vi "AIs-Freq_CA.vi"(5 "下限值":dbl=1.7 format="%#_13g", 6 "Slot":T1, 7 "上限值":dbl=3.0 format="%#_13g", 8 "error in":errorcluster, 9 "循环次数":i32=10, 10 "Mode":string, 11 "CHs":string[](array[string])) -> (0 "error out":errorcluster, 1 "幅值":dbl caption="检测到的幅值" format="%.2p", 2 "RMS value":dbl caption="均方根值" format="%0.2p", 3 "波形图":waveform(dbl)[](graph), 4 "Strout":string)   [LabVIEW 2013]
uses:
  SystemCode/SysControl/Slot.ctl
  <vilib>/Analysis/3filter.llb/Filter Passband Type.ctl
  <vilib>/DAQmx/read.llb/DAQmx Read (Analog 1D Wfm NChan NSamp).vi
  SourceCode/GlobalValue.vi
  <vilib>/DAQmx/create/channels.llb/DAQmx Create Channel (AI-Voltage-Basic).vi
  <vilib>/DAQmx/configure/timing.llb/DAQmx Timing (Sample Clock).vi
  <vilib>/Analysis/3filter.llb/Butterworth Filter (DBL).vi
  <vilib>/measure/matone.llb/Extract Single Tone Information 1 Chan.vi
  <vilib>/measure/matone.llb/SINAD Analyzer 1 Chan.vi
  <vilib>/measure/madcrms.llb/Basic Averaged DC-RMS for 1 Chan.vi
  <vilib>/DAQmx/miscellaneous.llb/DAQmx Fill In Error Info.vi
  <vilib>/measure/NI_MAPro.lvlib
  <vilib>/Analysis/NI_AALBase.lvlib
panel:
  out "THD Plus Noise":dbl caption="总谐波失真叠加噪声" format="%.2p"
  out "SINAD (dB)":dbl format="%.2p"
  # "ASelfTest"
  # "Audio"
  # "Audio"
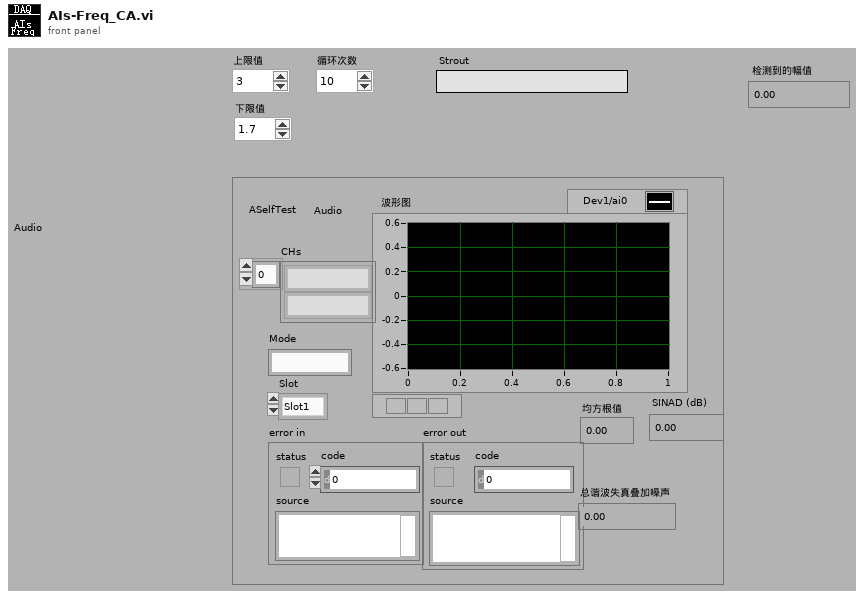
[diagram p1: front panel]
types:
  T1 = typedef "Slot.ctl" = enum16{"Slot1", "Slot2", "Slot3", "Slot4"}
  T2 = typedef "NI_AALBase.lvlib/Filter Passband Type.ctl" = enum32{"Lowpass", "Highpass", "Bandpass", "Bandstop"}
  T3 = typedef "DAQConfig.ctl" = cluster{"DIO":string[][], "AO":string[][], "AI":string[][]}
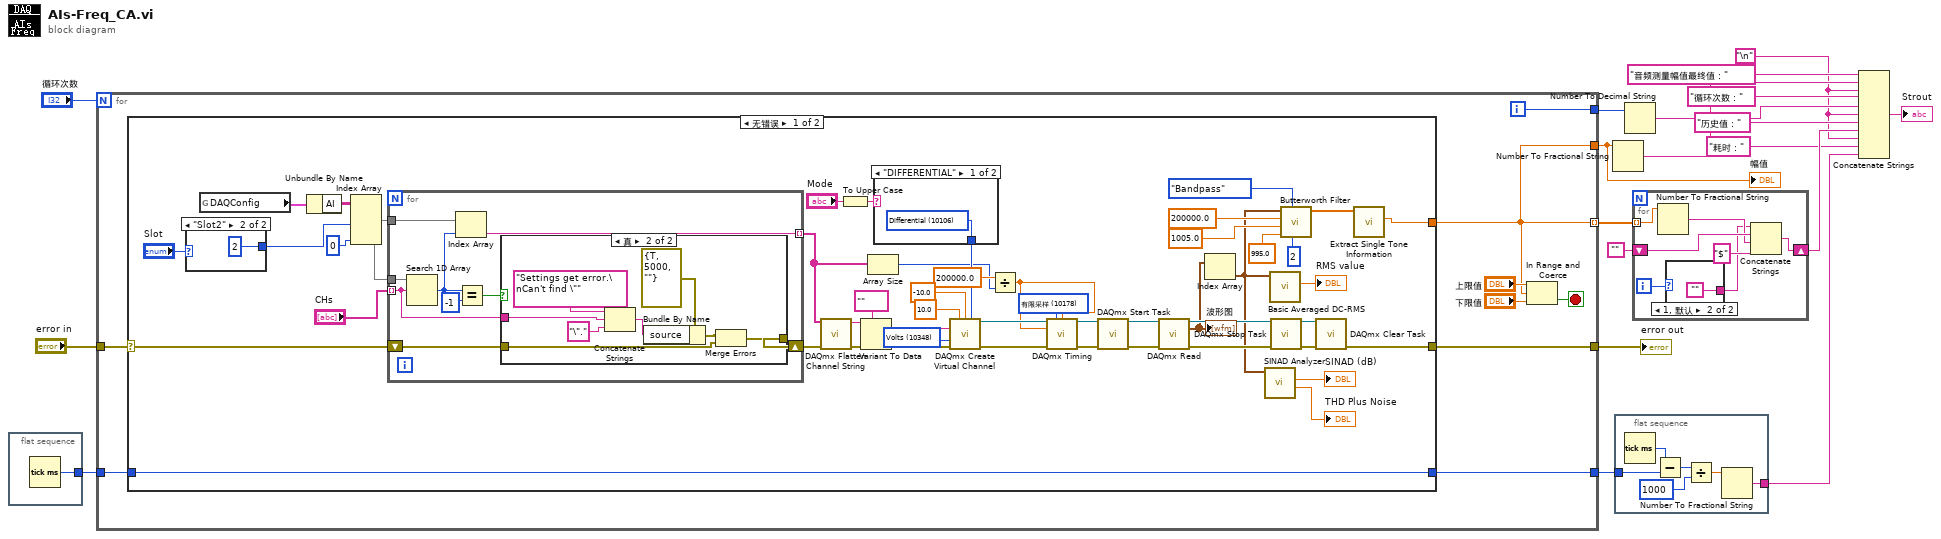
[diagram p0: block diagram]
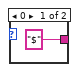
[diagram p2: hidden frame]
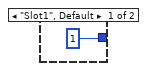
[diagram p3: hidden frame]
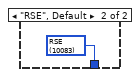
[diagram p5: hidden frame]
diagram:
  w5 = "\n"
  n1 = flat-sequence {
    tunnel: [w20] -> w18
    frame #0 {
      n2 = Tick Count (ms)() -> (millisecond timer value=w20:u32)
    }
  }
  n3 = for {
    N: "循环次数" -> [_]
    tunnel: [w22] -> w9 mode=indexing
    tunnel: w18 -> [w29]
    tunnel: [w28] -> w17
    tunnel: [w24] -> w16
    tunnel: "error in" -> [w23]
    tunnel: [w22] -> w1
    tunnel: [w21] -> w11
    i -> [w21]
    stop <- w27 stop-if-true
    n4 = case shown="无错误" w23 {
      selector: w23 -> [w63 w103]
      tunnel: [w79 w103] -> w24
      tunnel: [w38 _] -> w22
      tunnel: w29 -> [w37 w102]
      tunnel: [w37 w102] -> w28
      frame No Error {
        w59 = 10178 items=["有限采样"=10178, "连续采样"=10123, "硬件定时单点"=12522] ("sample mode")
        w74 = 10348 items=["Volts"=10348, "From Custom Scale"=10065] ("units")
        n5 = case shown="\"Slot2\"" "Slot" {
          tunnel: [1 ("索引 (行)") 2 ("索引 (行)")] -> w45
          frame "Slot1", Default {
          }
          frame "Slot2" {
          }
        }
        n6 = global read "GlobalValue.vi" "DAQConfig"() -> (w43:T3)
        n7 = Unbundle By Name(w43) -> ("AI"=w70:string[][])
        n8 = Index Array(array=w70, index (col) #1=w45, index (col) #2=0 ("索引 (列)")) -> (element #1=w68:string[], element #2=w67:string[])  [unwired: 2 in]
        n9 = for {
          tunnel: w68 -> [w88]
          tunnel: w67 -> [w87]
          tunnel: "CHs" -> [w85] mode=indexing
          tunnel: [w82] -> w49 mode=indexing
          shift-right: [w84] -> w51
          shift-left: w63 -> [w83]
          n10 = Search 1D Array(1D array=w87, element=w85) -> (index of element=w90:i32)  [unwired: 1 in]
          n11 = Index Array(array=w88, index=w90) -> (element=w82:string)
          n12 = Equal?(x=w90, y=-1) -> (x = y?=w86:bool)
          n13 = case shown="真" w86 {
            tunnel: w83 -> [w91 w95]
            tunnel: [w91 w94] -> w84
            tunnel: w85 -> [_ w93]
            frame False {
            }
            frame True {
              n14 = Concatenate Strings("Settings get error.\nCan't find \"" ("message"), w93, "\"." ("string")) -> (w98:string)
              n15 = Bundle By Name(cluster=errorcluster {"status"=TRUE, "code"=5000, "source"=""} ("error in 1 (no error)"), "source"=w98) -> (w97:errorcluster)
              n16 = Merge Errors(w97, w95) -> (w94:errorcluster)
            }
          }
        }
        n17 = call <vilib>:"DAQmx Flatten Channel String.vi"("names in"=w49, "error in"=w51) -> ("names out"=w50:string, "error out"=w52:errorcluster)  [unwired: 12 in]
        n18 = To Upper Case(1:"Mode") -> (0:w61:string)
        n19 = Variant To Data(error in=w52, type=tag "" ("lines"), Variant=w50) -> (data=w65:tag, error out=w64:errorcluster)
        n20 = Array Size(array=w49) -> (size(s)=w47:i32)
        n21 = case shown="\"DIFFERENTIAL\"" w61 {
          tunnel: [w100 w101] -> w60
          frame "DIFFERENTIAL" {
            w100 = 10106 items=["default"=-1, "RSE"=10083, "NRSE"=10078, "Differential"=10106, "Pseudodifferential"=12529] ("input terminal configuration")
          }
          frame "RSE", Default {
            w101 = 10083 items=["default"=-1, "RSE"=10083, "NRSE"=10078, "Differential"=10106, "Pseudodifferential"=12529] ("input terminal configuration")
          }
        }
        n22 = call-poly <vilib>:"DAQmx Create Virtual Channel.vi"("maximum value"=10.0, "minimum value"=-10.0, "input terminal configuration"=w60, "physical channels"=w65, "units"=w74, "error in"=w64) -> ("task out"=w58:refnum<k21>, "error out"=w56:errorcluster)  [unwired: 8 in]
        n23 = Divide(x=200000.0, y=w47) -> (x/y=w44:dbl)
        n24 = call-poly <vilib>:"DAQmx Timing.vi"("task/channels in"=w58, "sample mode"=w59, "samples per channel"=w44, "rate"=w44, "error in"=w56) -> ("task out"=w57:refnum<k21>, "error out"=w55:errorcluster)  [unwired: 2 in, 7 out]
        n25 = call <vilib>:"DAQmx Start Task.vi"("task/channels in"=w57, "error in"=w55) -> ("task out"=w78:refnum<k21>, "error out"=w77:errorcluster)  [unwired: 12 in]
        n26 = call-poly <vilib>:"DAQmx Read.vi"("task/channels in"=w78, "error in"=w77) -> ("task out"=w73:refnum<k21>, "data"=w42:waveform(dbl)[], "error out"=w54:errorcluster)  [unwired: 11 in]
        "波形图" <- w42
        n27 = Index Array(array=w42) -> (element=w31:waveform(dbl))  [unwired: 1 in]
        n28 = call-poly <vilib>:"SINAD Analyzer.vi"("signal in"=w31) -> ("THD Plus Noise"=→"THD Plus Noise":dbl, "SINAD (dB)"=→"SINAD (dB)":dbl)  [unwired: 5 in, 4 out]
        n29 = call-poly <vilib>:"Basic Averaged DC-RMS.vi"("signal in"=w31) -> ("RMS value"=→"RMS value":dbl)  [unwired: 7 in, 3 out]
        n30 = call <vilib>:"DAQmx Stop Task.vi"("task/channels in"=w73, "error in"=w54) -> ("task out"=w76:refnum<k21>, "error out"=w75:errorcluster)  [unwired: 12 in]
        n31 = call-poly <vilib>:"Butterworth Filter.vi"("order"=2, "filter type"=Filter_Passband_Type."Bandpass", "low cutoff freq: fl"=995.0, "high cutoff freq: fh"=1005.0, "sampling freq: fs"=200000.0, "X"=w31) -> ("Filtered X"=w30:dbl[])  [unwired: 2 in, 1 out]
        n32 = call <vilib>:"DAQmx Clear Task.vi"("task in"=w76, "error in"=w75) -> ("error out"=w79:errorcluster)  [unwired: 13 in]
        n33 = call-poly <vilib>:"Extract Single Tone Information.vi"("time signal in"=w30) -> ("detected amplitude"=w38:dbl)  [unwired: 5 in, 5 out]
      }
      frame Error {
      }
    }
    n34 = In Range and Coerce(upper limit="上限值", x=w22, lower limit="下限值") -> (In Range?=w27:bool)  [unwired: 1 out]
  }
  "error out" <- w16
  "幅值" <- w1
  n35 = Number To Fractional String(number=w1) -> (F-format string=w13:string)  [unwired: 3 in]
  n36 = flat-sequence {
    tunnel: w17 -> [w108]
    tunnel: [w104] -> w3
    frame #0 {
      n37 = Tick Count (ms)() -> (millisecond timer value=w109:u32)
      n38 = Subtract(x=w109, y=w108) -> (x-y=w106:u32)
      n39 = Divide(x=w106, y=u32 1000) -> (x/y=w105:dbl)
      n40 = Number To Fractional String(number=w105) -> (F-format string=w104:string)  [unwired: 3 in]
    }
  }
  n41 = Number To Decimal String(number=w11) -> (decimal integer string=w10:string)  [unwired: 1 in]
  n42 = for {
    tunnel: w9 -> [w116] mode=indexing
    shift-right: [w112] -> w6
    shift-left: "" -> [w115]
    i -> [w111]
    n43 = Number To Fractional String(number=w116) -> (F-format string=w114:string)  [unwired: 3 in]
    n44 = case shown="1, 默认" w111 {
      tunnel: ["$" ""] -> w110
      frame 0 {
      }
      frame 1, Default {
      }
    }
    n45 = Concatenate Strings(w110, w115, w114, "$") -> (w112:string)
  }
  n46 = Concatenate Strings("音频测量幅值最终值：", w13, w5, "循环次数：", w10, w5, "历史值：", w6, w5, "耗时：", w3) -> (→"Strout":string)
